vi "HOL_SWERVE_KINEMATIC_FGV.vi"(9 "in SWERVE_DRIVE_KINEMATICS":T1 {"PrevCoR"."Y" format="%14.3f"; "PrevCoR"."X" format="%14.3f"; "Modules"."Y" format="%14.3f"; "Modules"."X" format="%14.3f"}, 11 "WRITE":bool) -> (1 "out SWERVE_DRIVE_KINEMATICS":T1 {"PrevCoR"."Y" format="%14.3f"; "PrevCoR"."X" format="%14.3f"; "Modules"."Y" format="%14.3f"; "Modules"."X" format="%14.3f"})   [LabVIEW 2019]
uses:
  <vilib>/Rock Robotics/WPI/ThirdParty/JAS_Junk/TrajLib/SWERVE_DRIVE_KINEMATICS.ctl
  <vilib>/Analysis/Matrix/Datatypes/RealMatrix.ctl
  <vilib>/Rock Robotics/WPI/ThirdParty/JAS_Junk/TrajLib/TRANSLATION2D.ctl
  <vilib>/Rock Robotics/WPI/ThirdParty/JAS_Junk/TrajLib/Trajectory_Library.lvlib
  <vilib>/Analysis/Matrix/NI_Matrix.lvlib
panel:
  # "This is purposefully \n\nNOT re-entrant."
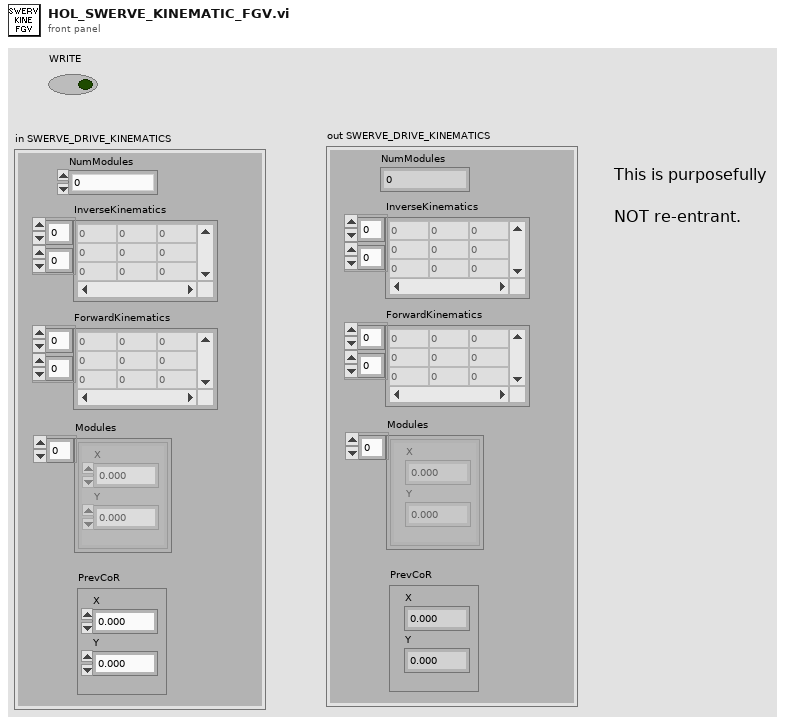
[diagram p1: front panel]
types:
  T1 = typedef "Trajectory_Library.lvlib/SWERVE_DRIVE_KINEMATICS.ctl" = cluster{"NumModules":i32, "InverseKinematics":T2, "ForwardKinematics":T2, "Modules":T3[], "PrevCoR":T3}
  T2 = typedef "NI_Matrix.lvlib/RealMatrix.ctl" = dbl[][]
  T3 = typedef "Trajectory_Library.lvlib/TRANSLATION2D.ctl" = cluster{"X":dbl, "Y":dbl}
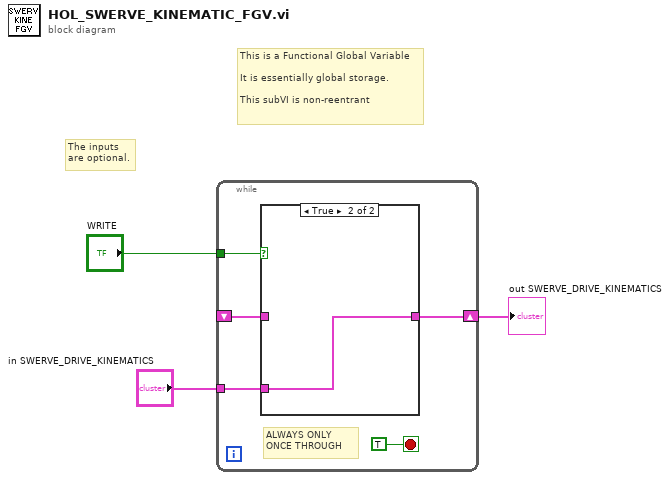
[diagram p0: block diagram]
diagram:
  # "The inputs \nare optional."
  # "This is a Functional Global Variable\n\nIt is essentially global storage.\n\nThis subVI is non-reentrant"
  n1 = while {
    shift-right: [w6] -> w2
    shift-left: _ -> [w4]
    tunnel: "WRITE" -> [w7]
    tunnel: "in SWERVE_DRIVE_KINEMATICS" -> [w5]
    stop <- TRUE stop-if-true
    # "ALWAYS ONLY\nONCE THROUGH"
    n2 = case shown="True" w7 {
      tunnel: [w9 w10] -> w6
      tunnel: w5 -> [_ w10]
      tunnel: w4 -> [w9 _]
      frame False {
      }
      frame True {
      }
    }
  }
  "out SWERVE_DRIVE_KINEMATICS" <- w2
